vi "UsingTheOtherLEDs.vi"() -> ()   [LabVIEW 2012]
panel:
  in  "LED3":bool
  in  "LED2":bool
  in  "LED1":bool
  in  "LED0":bool
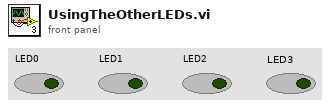
[diagram p1: front panel]
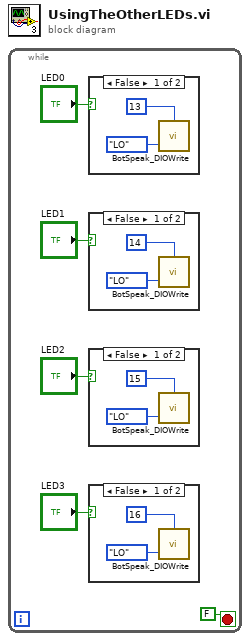
[diagram p0: block diagram]
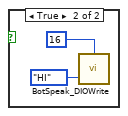
[diagram p2: hidden frame]
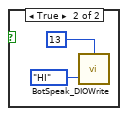
[diagram p3: hidden frame]
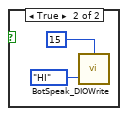
[diagram p4: hidden frame]
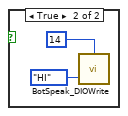
[diagram p5: hidden frame]
diagram:
  n1 = while {
    stop <- FALSE stop-if-true
    n2 = case shown="False" "LED0" {
      frame False {
        n3 = call <userlib>:"BotSpeak_DIOWrite.vi"("State"=enum32{"LO", "HI"}."LO", "DIO Line"=u32 13) -> ()  [unwired: 1 in, 2 out]
      }
      frame True {
        n4 = call <userlib>:"BotSpeak_DIOWrite.vi"("State"=enum32{"LO", "HI"}."HI", "DIO Line"=u32 13) -> ()  [unwired: 1 in, 2 out]
      }
    }
    n5 = case shown="False" "LED1" {
      frame False {
        n6 = call <userlib>:"BotSpeak_DIOWrite.vi"("State"=enum32{"LO", "HI"}."LO", "DIO Line"=u32 14) -> ()  [unwired: 1 in, 2 out]
      }
      frame True {
        n7 = call <userlib>:"BotSpeak_DIOWrite.vi"("State"=enum32{"LO", "HI"}."HI", "DIO Line"=u32 14) -> ()  [unwired: 1 in, 2 out]
      }
    }
    n8 = case shown="False" "LED2" {
      frame False {
        n9 = call <userlib>:"BotSpeak_DIOWrite.vi"("State"=enum32{"LO", "HI"}."LO", "DIO Line"=u32 15) -> ()  [unwired: 1 in, 2 out]
      }
      frame True {
        n10 = call <userlib>:"BotSpeak_DIOWrite.vi"("State"=enum32{"LO", "HI"}."HI", "DIO Line"=u32 15) -> ()  [unwired: 1 in, 2 out]
      }
    }
    n11 = case shown="False" "LED3" {
      frame False {
        n12 = call <userlib>:"BotSpeak_DIOWrite.vi"("State"=enum32{"LO", "HI"}."LO", "DIO Line"=u32 16) -> ()  [unwired: 1 in, 2 out]
      }
      frame True {
        n13 = call <userlib>:"BotSpeak_DIOWrite.vi"("State"=enum32{"LO", "HI"}."HI", "DIO Line"=u32 16) -> ()  [unwired: 1 in, 2 out]
      }
    }
  }
